vi "Send Program Text to Notebook.vi"(8 "Error In":errorcluster, 9 "Text (none)":string, 10 "Text Format (Message)":T1, 11 "Notebook Queue in":refnum<queue>) -> (0 "Error Out":errorcluster)   [LabVIEW 2021, in "Notebook.lvlib"]
doc: "Sends the <B>Text</B> to the Notebook (whose <b>Notebook Queue</B> need to be provided), bracketted by to 'New Line' (\\n) characters.\n\nThe user can provide an optional <B>Text Format</B> (defualt: 'Message').\n\nThe current Theme is used."
uses:
  Notebook.lvlib
  Rich Text Box/Text Format List.ctl
  Notebook Action Q Element.ctl
  Notebook Action List.ctl
  Rich Text Box/Formatted Text.ctl
  Rich Text Box/Text Formatting.ctl
  Rich Text Box/Text Colors.ctl
  Rich Text Box/Text Style.ctl
  Rich Text Box/Text Alignment.ctl
  Rich Text Box/Rich Text Box.lvlib
panel:
  # "see the License on the block diagram (Ctrl+E or Window:Show Block Diagram)"
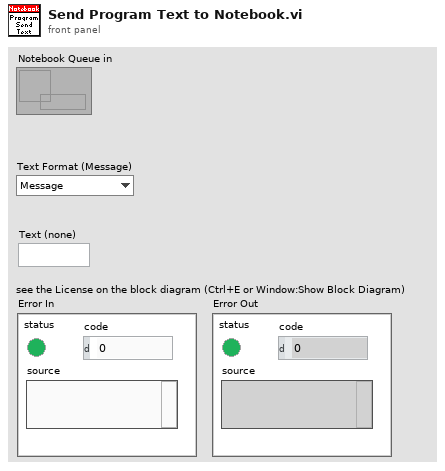
[diagram p1: front panel]
types:
  T1 = typedef "Notebook.lvlib/Text Format List.ctl" = enum16{"Message", "Result", "Error", "Setting", "Verbose", "Warning"}
  T2 = typedef "Notebook.lvlib/Notebook Action Q Element.ctl" = cluster{"Action":T3, "Variant":variant}
  T3 = typedef "Notebook.lvlib/Notebook Action List.ctl" = enum16{"Idle", "Init", "Check Content Change", "User added content", "Program added text", "Program added Picture ", "Save Notebook", "Quit", "Open", "Close", "Update Window Title", "Edit Text Styles", "Update Theme", "Save Themes", "Load Themes"}
  T4 = typedef "Rich Text Box.lvlib/Formatted Text.ctl" = cluster{"Text":string, "Text Formatting":T5}
  T5 = typedef "Rich Text Box.lvlib/Text Formatting.ctl" = cluster{"Font":string, "Text Color":T6, "Background Color":T6, "Style":T7, "Font Size":dbl, "Alignment":T8}
  T6 = typedef "Rich Text Box.lvlib/Text Colors.ctl" = enum16{"Unchanged", "Black", "Blue", "Cyan", "Maroon", "Gray", "Violet", "Green", "Light Green", "Orange", "Yellow", "Magenta", "Red", "White"}
  T7 = typedef "Rich Text Box.lvlib/Text Style.ctl" = enum16{"Regular", "Bold", "Italic", "Underline", "Strikeout"}
  T8 = typedef "Rich Text Box.lvlib/Text Alignment.ctl" = enum16{"Left", "Right", "Center"}
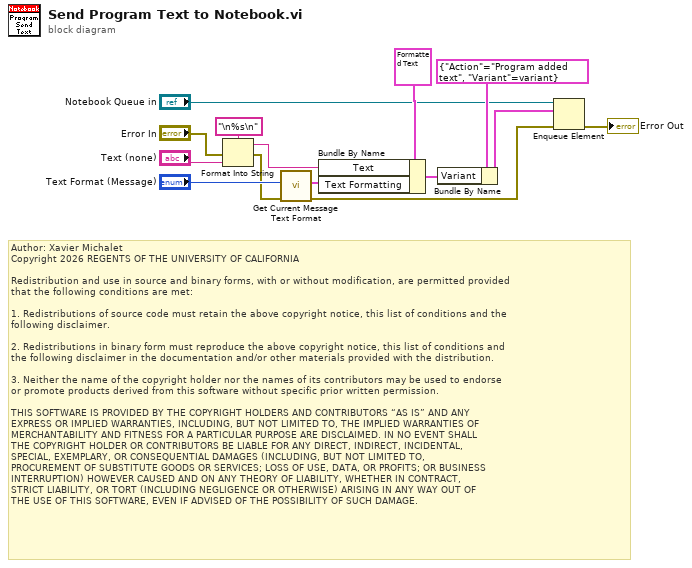
[diagram p0: block diagram]
diagram:
  # "Author: Xavier Michalet\nCopyright 2026 REGENTS OF THE UNIVERSITY OF CALIFORNIA\n\nRedistribution and use in source and binary forms, with or without modification, are permitted provided\nthat the following conditions are met:\n\n1. Redistributions of source code must retain the above copyright notice, this list of conditions and the\nfollowing disclaimer.\n\n2. Redistributions in binary form must reproduce the above copyright notice, this list of conditions and\nthe following disclaimer in the documentation and/or other materials provided with the distribution.\n\n3. Neither the name of the copyright holder nor the names of its contributors may be used to endorse \nor promote products derived from this software without specific prior written permission.\n\nTHIS SOFTWARE IS PROVIDED BY THE COPYRIGHT HOLDERS AND CONTRIBUTORS “AS IS” AND ANY \nEXPRESS OR IMPLIED WARRANTIES, INCLUDING, BUT NOT LIMITED TO, THE IMPLIED WARRANTIES OF\nMERCHANTABILITY AND FITNESS FOR A PARTICULAR PURPOSE ARE DISCLAIMED. IN NO EVENT SHALL\nTHE COPYRIGHT HOLDER OR CONTRIBUTORS BE LIABLE FOR ANY DIRECT, INDIRECT, INCIDENTAL, \nSPECIAL, EXEMPLARY, OR CONSEQUENTIAL DAMAGES (INCLUDING, BUT NOT LIMITED TO, \nPROCUREMENT OF SUBSTITUTE GOODS OR SERVICES; LOSS OF USE, DATA, OR PROFITS; OR BUSINESS\nINTERRUPTION) HOWEVER CAUSED AND ON ANY THEORY OF LIABILITY, WHETHER IN CONTRACT, \nSTRICT LIABILITY, OR TORT (INCLUDING NEGLIGENCE OR OTHERWISE) ARISING IN ANY WAY OUT OF\nTHE USE OF THIS SOFTWARE, EVEN IF ADVISED OF THE POSSIBILITY OF SUCH DAMAGE."
  n1 = Format Into String(format string="\n%s\n", error in="Error In", "Text (none)") -> (resulting string=w3:string, error out=w1:errorcluster)  [unwired: 1 in]
  n2 = call "Get Current Message Text Format.vi"("Error In"=w1, "Text Format"="Text Format (Message)") -> ("Error Out"=w7:errorcluster, "Message Formatting"=w14:T5)  [unwired: 7 in]
  n3 = Bundle By Name(cluster=T4 {"Text"="", "Text Formatting"={"Font"="", "Text Color"=enum."Unchanged", "Background Color"=enum."Unchanged", "Style"=enum."Regular", "Font Size"=-1.0, "Alignment"=enum."Left"}} ("Formatted Text"), "Text"=w3, "Text Formatting"=w14) -> (w13:T4)
  n4 = Bundle By Name(cluster=T2 {"Action"=enum."Program added text", "Variant"=variant} ("element"), "Variant"=w13) -> (w11:T2)
  n5 = Enqueue Element(queue="Notebook Queue in", element=w11, error in (no error)=w7) -> (error out=→"Error Out":errorcluster)  [unwired: 1 in, 2 out]
